vi "FSK_DeSync.vi"(8 "error in (no error)":errorcluster caption="错误输入（无错误）", 10 "RecvSymbolSampled":dbl[](array[numeric]), 11 "PathIn":path) -> (0 "error out":errorcluster caption="错误输出", 2 "RecvDeSync":dbl[](array[numeric]) format="%#_13g", 3 "PathOut":path)   [LabVIEW 2015]
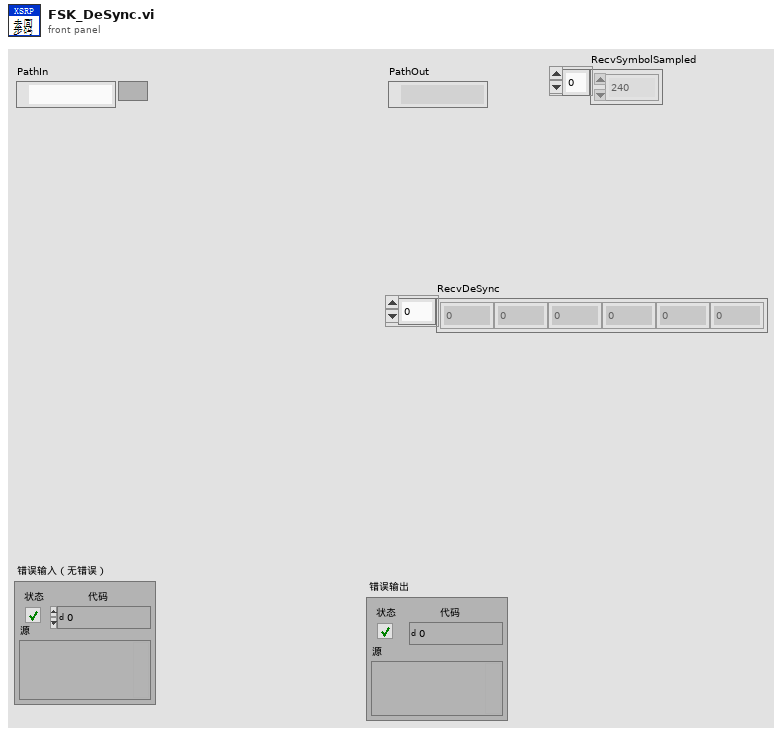
[diagram p1: front panel]
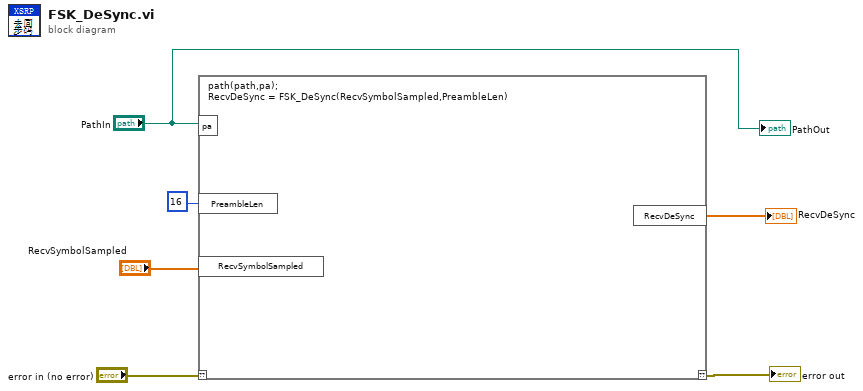
[diagram p0: block diagram]
diagram:
  n1 = script code="path(path,pa);\nRecvDeSync = FSK_DeSync(RecvSymbolSampled,PreambleLen)"("??"="error in (no error)", "pa"="PathIn", "RecvSymbolSampled"="RecvSymbolSampled", "PreambleLen"=16) -> ("??"=→"error out":errorcluster, "RecvDeSync"=→"RecvDeSync":dbl[])
  "PathOut" <- "PathIn"
